vi "New-Engine.vi"(8 "error in (no error)":errorcluster) -> (0 "error out":errorcluster, 3 "Engine":refnum<class "Engine.lvclass">)   [LabVIEW 2020, in "GLF.lvlib" / "Engine.lvclass"]
uses:
  Engine.lvclass
  IAmGLF/IAmGLF.lvclass
  Core.vi
  Engine.lvclass/Engine.ctl
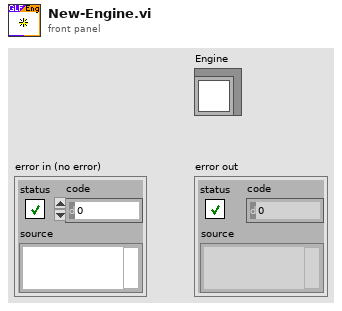
[diagram p1: front panel]
types:
  T1 = cluster{"Engine":refnum<class "IAmGLF.lvclass">, "Error":errorcluster}
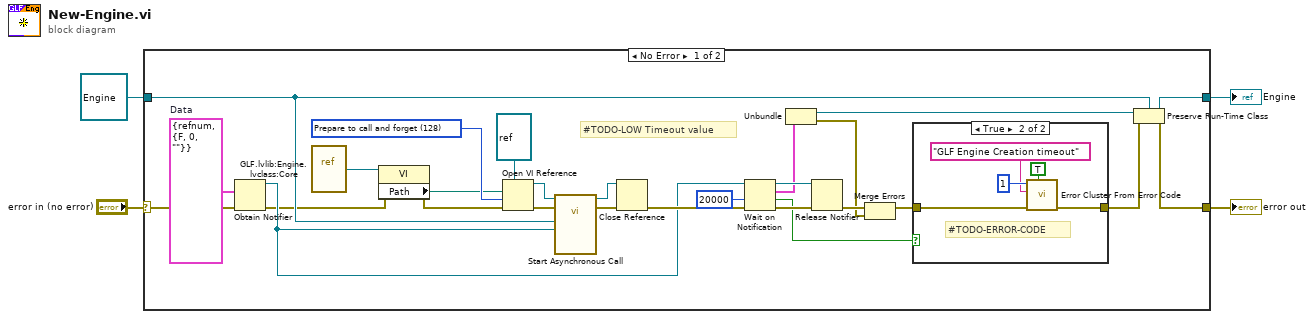
[diagram p0: block diagram]
diagram:
  n1 = case shown="No Error" "error in (no error)" {
    selector: "error in (no error)" -> [w28 w39]
    tunnel: [w27 w39] -> w3
    tunnel: [w18 w38] -> w1
    tunnel: refnum<class "Engine.lvclass"> refnum ("Engine in") -> [w17 w38]
    frame No Error {
      w12 = T1 {"Engine"=refnum, "Error"={"status"=FALSE, "code"=0, "source"=""}}  # Data
      w21 = 128 items=["Record modifications"=1, "Open templates for editing"=2, "Prompt user to save"=4, "Prepare for reentrant run"=8, "Prompt to find missing subVIs"=16, "Hide loading dialog box"=32, "Enable simultaneous calls"=64, "Prepare to call and forget"=128, "Simultaneous call and forget"=192, "Prepare to call and collect"=256, "Simultaneous call and collect"=320]
      # "#TODO-LOW Timeout value"
      n2 = Obtain Notifier(notification data type=w12, error in (no error)=w28) -> (notifier out=w19:refnum<notifier>, error out=w14:errorcluster)  [unwired: 2 in, 1 out]
      n3 = vi-ref "GLF.lvlib:Engine.lvclass:Core.vi"() -> (w16:refnum<vi>)
      n4 = property class="VI"(reference=w16, error in=w14) -> (error out=w13:errorcluster, "Path"=w15:path)  [unwired: 1 out]
      n5 = Open VI Reference(type specifier VI Refnum (for type only)=refnum<vi> refnum, vi path=w15, options=w21, error in (no error)=w13) -> (vi reference=w24:refnum<vi>, error out=w26:errorcluster)  [unwired: 2 in]
      n6 = call-by-ref "Start Asynchronous Call"(reference=w24, error in=w26, "Class Return Notifier"=w19, "Engine in"=w17) -> (reference out=w23:refnum<vi>, error out=w25:errorcluster)  [unwired: 10 in]
      n7 = Close Reference(reference=w23, error in (no error)=w25) -> (error out=w20:errorcluster)
      n8 = Wait on Notification(notifier=w19, timeout in ms (-1)=20000, error in (no error)=w20) -> (notifier out=w31:refnum<notifier>, notification=w11:T1, timed out?=w5:bool, error out=w30:errorcluster)  [unwired: 1 in]
      n9 = Unbundle(w11) -> ("Engine"=w10:refnum<class "IAmGLF.lvclass">, "Error"=w8:errorcluster)
      n10 = Release Notifier(notifier=w31, error in (no error)=w30) -> (error out=w29:errorcluster)  [unwired: 1 in, 2 out]
      n11 = Merge Errors(w29, w8) -> (w9:errorcluster)
      n12 = case shown="True" w5 {
        tunnel: w9 -> [w32 w37]
        tunnel: [w32 w36] -> w6
        frame False {
        }
        frame True {
          # "#TODO-ERROR-CODE"
          n13 = call <vilib>:"Error Cluster From Error Code.vi"("show call chain? (False)"=TRUE, "error in (no error)"=w37, "error message (\"\")"="GLF Engine Creation timeout" ("error message (\"\")"), "error code (0)"=1) -> ("error out"=w36:errorcluster)  [unwired: 5 in]
        }
      }
      n14 = Preserve Run-Time Class(object in=w10, error in=w6, 2:w17) -> (object out=w18:refnum<class "Engine.lvclass">, error out=w27:errorcluster)
    }
    frame Error {
    }
  }
  "error out" <- w3
  "Engine" <- w1
